vi "TriangleMessage.vi"(0 "Frequency":dbl, 1 "OutputStage":T2, 5 "Amplitude":dbl, 7 "Phase":dbl, 9 "Offset":dbl, 11 "Width":dbl, 12 "Filter":T1=enum."NoFilter") -> (4 "TriangleSignalMessage":string)   [LabVIEW 2019]
uses:
  OutputStageTypeDef.ctl
  FilterTypeDef.ctl
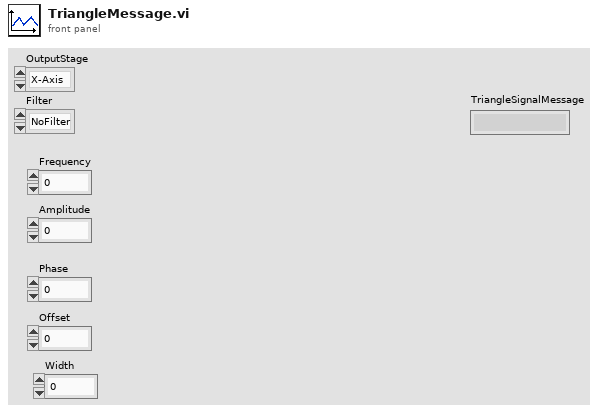
[diagram p1: front panel]
types:
  T1 = typedef "FilterTypeDef.ctl" = enum16{"IIR_Slow", "IIR_Fast", "NoFilter", "Bessel6thOrder300"}
  T2 = typedef "OutputStageTypeDef.ctl" = enum16{"X-Axis", "Y-Axis"}
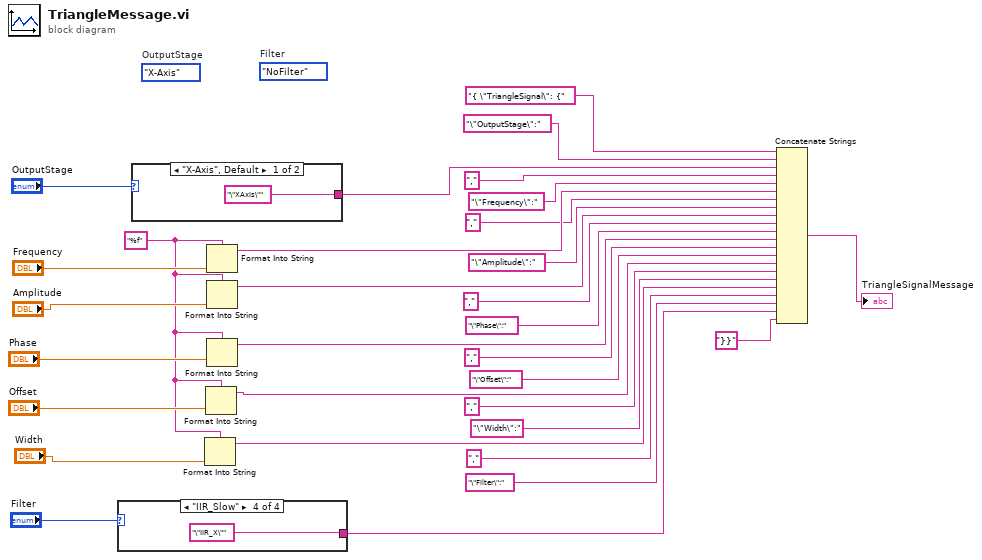
[diagram p0: block diagram]
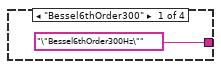
[diagram p2: hidden frame]
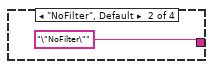
[diagram p3: hidden frame]
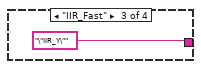
[diagram p4: hidden frame]
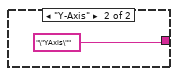
[diagram p5: hidden frame]
diagram:
  w7 = "%f" ("initial string")
  (unwired) FilterTypeDef."NoFilter"  # Filter
  (unwired) OutputStageTypeDef."X-Axis"  # OutputStage
  n1 = case shown="\"IIR_Slow\"" "Filter" {
    tunnel: ["\"Bessel6thOrder300Hz\"" "\"NoFilter\"" "\"IIR_Y\"" "\"IIR_X\""] -> w5
    frame "Bessel6thOrder300" {
    }
    frame "NoFilter", Default {
    }
    frame "IIR_Fast" {
    }
    frame "IIR_Slow" {
    }
  }
  n2 = case shown="\"X-Axis\", Default" "OutputStage" {
    tunnel: ["\"XAxis\"" "\"YAxis\""] -> w21
    frame "X-Axis", Default {
    }
    frame "Y-Axis" {
    }
  }
  n3 = Format Into String(format string=w7, "Width") -> (resulting string=w2:string)  [unwired: 2 in, 1 out]
  n4 = Format Into String(format string=w7, "Offset") -> (resulting string=w9:string)  [unwired: 2 in, 1 out]
  n5 = Format Into String(format string=w7, "Frequency") -> (resulting string=w18:string)  [unwired: 2 in, 1 out]
  n6 = Format Into String(format string=w7, "Amplitude") -> (resulting string=w15:string)  [unwired: 2 in, 1 out]
  n7 = Format Into String(format string=w7, "Phase") -> (resulting string=w12:string)  [unwired: 2 in, 1 out]
  n8 = Concatenate Strings("{ \"TriangleSignal\": {", "\"OutputStage\":", w21, ",", "\"Frequency\":", w18, ",", "\"Amplitude\":", w15, ",", "\"Phase\":", w12, ",", "\"Offset\":", w9, ",", "\"Width\":", w2, ",", "\"Filter\":", w5, "}}" ("string")) -> (→"TriangleSignalMessage":string)
